vi "3D Cartesian Coordinate Rotation (Euler).vi"   [LabVIEW 2017, in "NI_AALPro.lvlib"]
doc: "Rotates a three-dimensional Cartesian coordinate in the counterclockwise direction using the Euler angles method. Wire data to the <B>X</B> input to determine the polymorphic instance to use or manually select the instance."
uses:
  NI_AALPro.lvlib
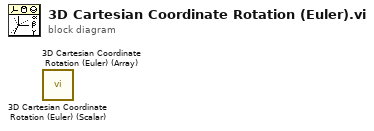
[diagram p0: block diagram]
diagram:
  n1 = call "3D Cartesian Coordinate Rotation (Euler) (Scalar).vi"() -> ()  [unwired: 8 in, 4 out]
  n2 = call "3D Cartesian Coordinate Rotation (Euler) (Array).vi"() -> ()  [unwired: 8 in, 4 out]
